vi "LED.vi"() -> ()   [LabVIEW 2019]
panel:
  in  "stop":bool
  in  "Knob":u8(knob) scale=50.0..1000.0
  in  "NB DE PAS":u8(slide) scale=-2.0..2.0
  out "?":bool[](array[boolean])
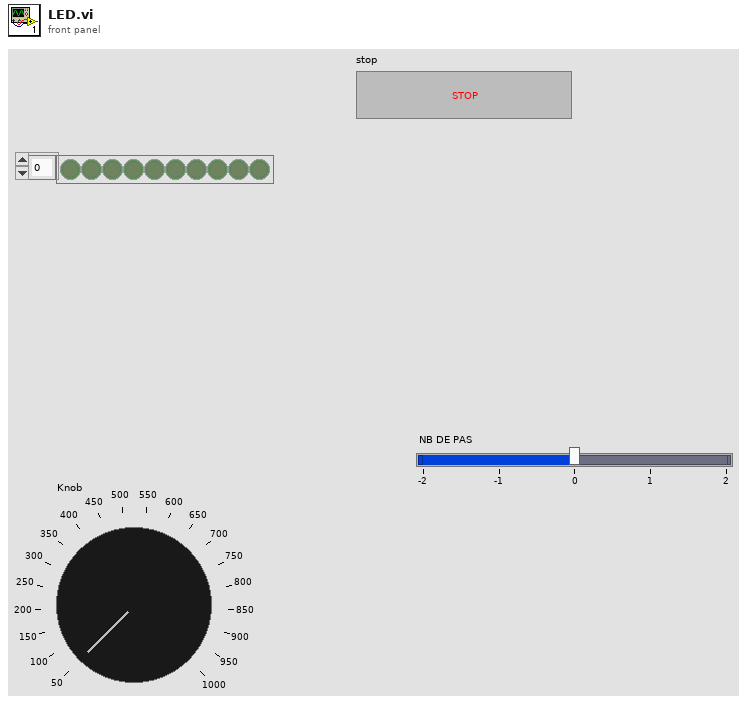
[diagram p1: front panel]
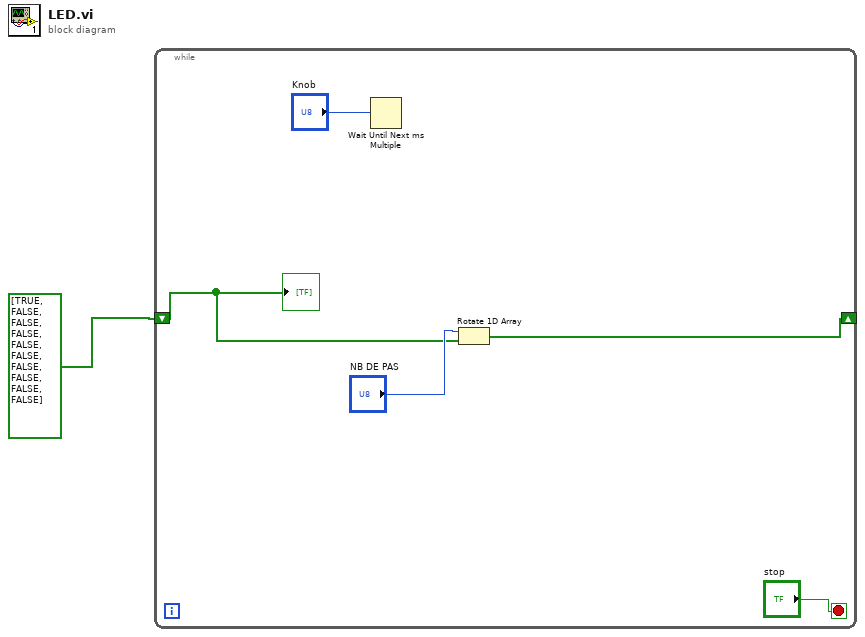
[diagram p0: block diagram]
diagram:
  n1 = while {
    shift-right: [w2] -> _
    shift-left: bool[] [TRUE, FALSE, FALSE, FALSE, FALSE, FALSE, FALSE, FALSE, FALSE, FALSE] -> [w3]
    stop <- "stop" stop-if-true
    n2 = Wait Until Next ms Multiple(millisecond multiple="Knob") -> ()  [unwired: 1 out]
    n3 = Rotate 1D Array(1:w3, 2:"NB DE PAS") -> (0:w2:bool[])
    "?" <- w3
  }
